vi "BC Test - Messages Only.vi"() -> ()   [LabVIEW 2016]
uses:
  Bus Controller/TypeDefs/Bus Controller Configuration.ctl
  Frames & Messages/TypeDefs/Message Config.ctl
  Frames & Messages/TypeDefs/Command Config.ctl
  Frames & Messages/TypeDefs/Message Control.ctl
  1553 SubComponent/TypeDefs/Parameter Table Data.ctl
  1553 SubComponent/TypeDefs/Scaling Information.ctl
  Frames & Messages/TypeDefs/RT-RT Message Config.ctl
  1553 Board/1553 Board.lvclass/1553 Board.ctl
  Bus Controller/Bus Controller.lvclass
  C:/SLSC 1553/Driver (Windows)/1553 SubComponent/1553 SubComponent.lvclass
  Frames & Messages/Message/Message.lvclass
  1553 Component/1553 Component.lvclass
  Frames & Messages/Major Frame/Major Frame.lvclass
  1553 Board/1553 Board.lvclass
  Utilities/FPGA Interface/FPGA Interface.lvclass
  SLSC 1553 API.lvlib
  1553 SubComponent/1553 SubComponent.lvclass
  Frames & Messages/RT-RT Message/RT-RT Message.lvclass
  C:/SLSC 1553/Driver (Windows)/Frames & Messages/Message/Message.lvclass
panel:
  in  "Inhibit Bus B":bool
  in  "Inhibit Bus A":bool
  in  "Scaled Data 2":dbl[](array[numeric])
  in  "Parameters 2":string[](array[string])
  in  "Update Param":bool
  out "Scaled Data":dbl[][](array[numeric])
  out "Parameters":string[][](array[string])
  out "error out":errorcluster
  in  "stop":bool
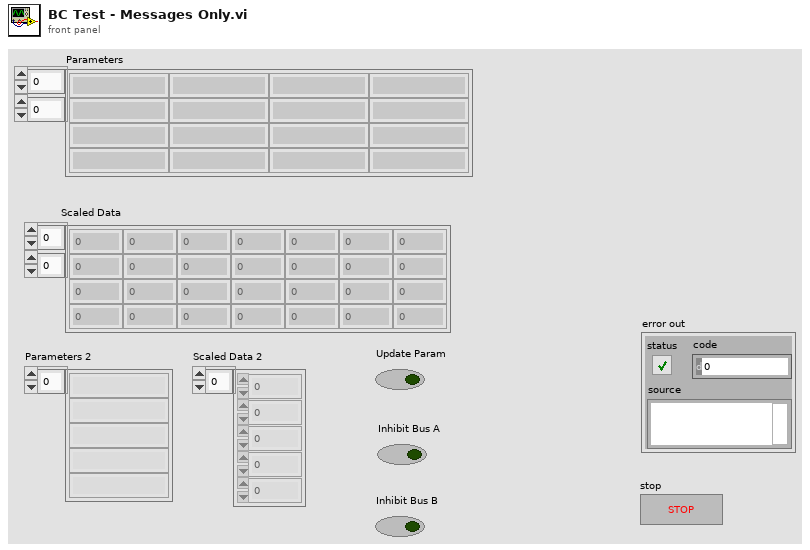
[diagram p1: front panel]
types:
  T1 = typedef "SLSC 1553 API.lvlib/RT-RT Message Config.ctl" = cluster{"Tx Command Config":T2}
  T2 = typedef "SLSC 1553 API.lvlib/Command Config.ctl" = cluster{"Command Type":enum16{"Transmit", "Receive"}, "Terminal Address (0-30)":u16, "SubAddress (1-30)":u16, "WC/MC (1-32)":u16, "Command Data":u16[]}
  T3 = typedef "SLSC 1553 API.lvlib/1553 SubComponent.lvclass/Parameter Table Data.ctl" = cluster{"Parameter Name":string, "Base Word":u16, "Address":u16, "Value":u64, "Mask":u16[], "Scaling Info":T4}
  T4 = typedef "SLSC 1553 API.lvlib/1553 SubComponent.lvclass/Scaling Information.ctl" = cluster{"Bit Offset":i32, "Bit Count":i32, "LSB Resolution":dbl, "2's Complement":bool, "Big Endian":bool}
  T5 = typedef "SLSC 1553 API.lvlib/Message Config.ctl" = cluster{"Time to Next Msg (100 us)":u16, "Command Config":T2, "Message Control":T6}
  T6 = typedef "SLSC 1553 API.lvlib/Message Control.ctl" = cluster{"MC17 Time Sync":bool, "Error Mask":bool, "Service Request Mask":bool, "Busy Mask":bool, "SubSystem Flag Mask":bool, "Terminal Flag Mask":bool, "Reserved Mask":bool, "Retry":bool, "Bus A / !Bus B":bool, "Self-Test Loopback":bool, "Broadcast Mask":bool, "EoM Interrupt":bool, "Mode Code Format":bool, "Broadcast Format":bool, "RT-RT Format":bool}
  T7 = typedef "SLSC 1553 API.lvlib/Bus Controller.lvclass/Bus Controller Configuration.ctl" = cluster{"BC Timeout":u16, "BC Retry":bool, "BC Second Retry":bool, "BC Retry Alt Bus":bool, "BC Second Retry Alt Bus":bool, "BC Retry on Status Bit":bool, "Msg Error No Data Valid":bool, "Busy Status No Data Valid":bool, "Msg Gap Timer":bool, "Watchdog Timer":bool, "Time Tag Sync":bool, "Even Time Tag Sync":bool, "Gap Check":bool, "Broadcast Mask Enable":bool}
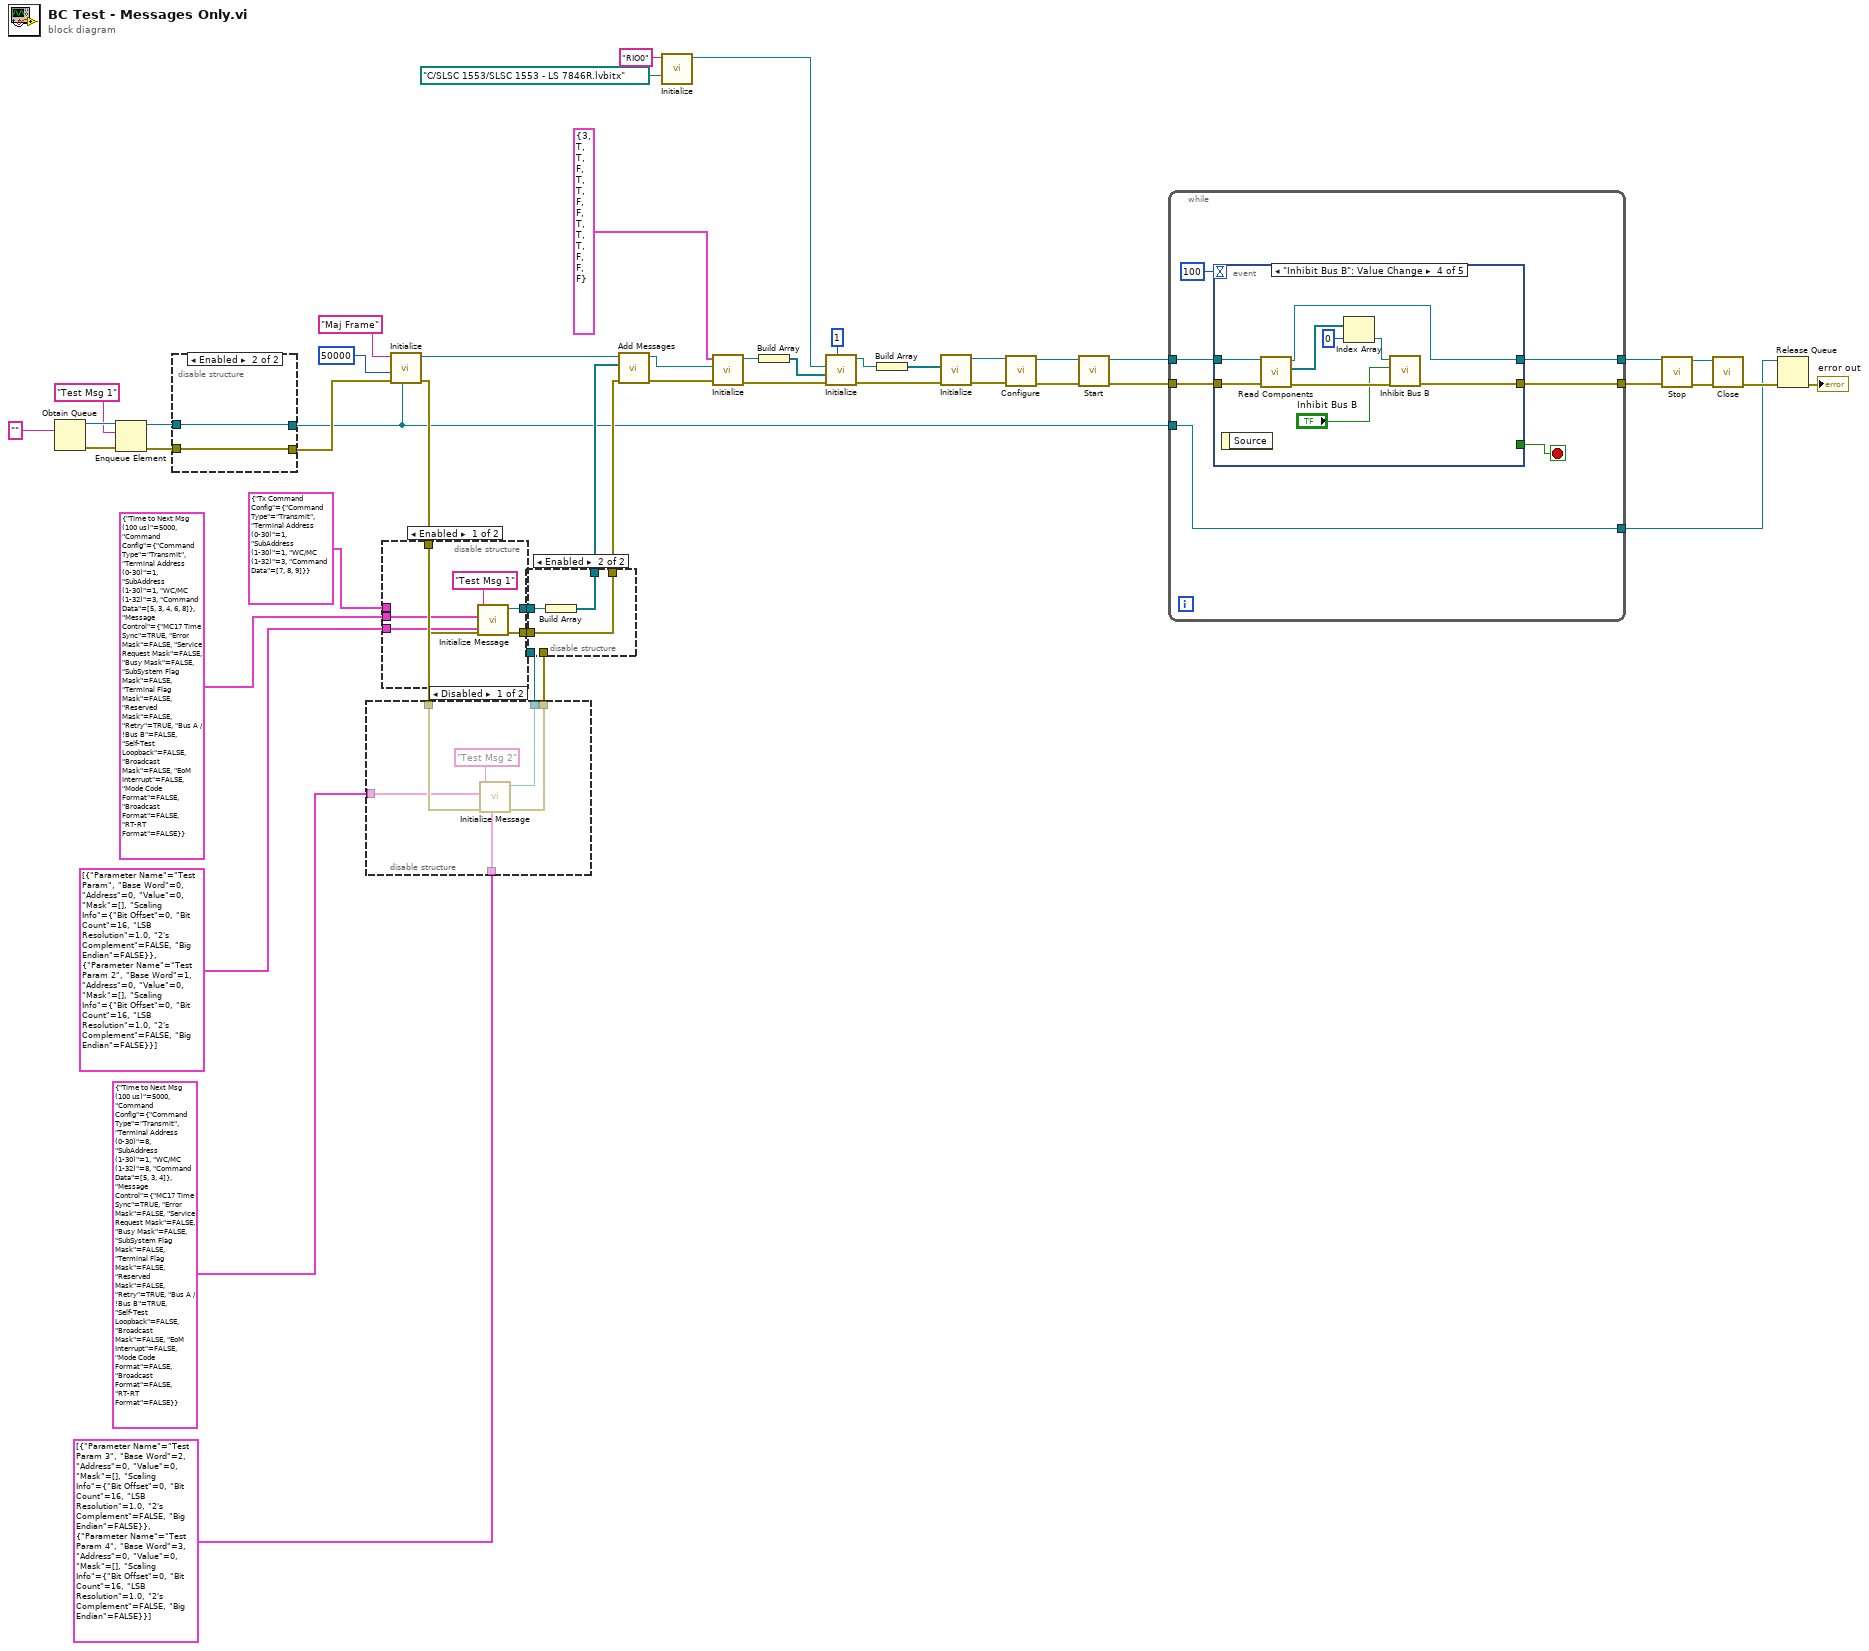
[diagram p0: block diagram]
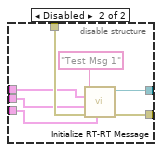
[diagram p2: hidden frame]
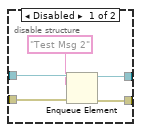
[diagram p3: hidden frame]
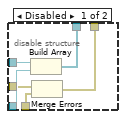
[diagram p4: hidden frame]
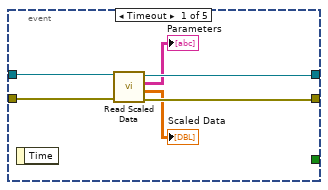
[diagram p6: hidden frame]
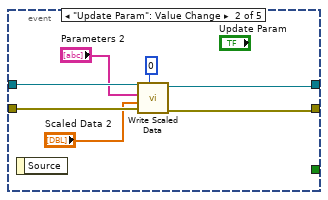
[diagram p7: hidden frame]
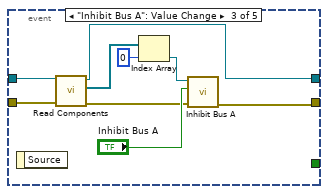
[diagram p8: hidden frame]
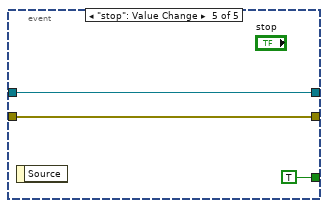
[diagram p9: hidden frame]
diagram:
  n1 = Obtain Queue(element data type="") -> (queue out=w46:refnum<queue>, error out=w47:errorcluster)  [unwired: 4 in, 1 out]
  n2 = Enqueue Element(queue=w46, element="Test Msg 1", error in (no error)=w47) -> (queue out=w44:refnum<queue>, error out=w45:errorcluster)  [unwired: 1 in, 1 out]
  n3 = disable-structure shown="Enabled" {
    disable-tunnel: w45 -> [w54 w55]
    disable-tunnel: w44 -> [w53 w56]
    disable-tunnel: [w51 w55] -> w42
    disable-tunnel: [w50 w56] -> w4
    frame Disabled {
      n4 = Enqueue Element(queue=w53, element="Test Msg 2", error in (no error)=w54) -> (queue out=w50:refnum<queue>, error out=w51:errorcluster)  [unwired: 1 in, 1 out]
    }
    frame Enabled {
    }
  }
  n5 = call "Initialize.vi"("Schedule"=w4, "error in (no error)"=w42, "Minor Frame Time (us)"=u16 50000, "ID"="Maj Frame") -> ("error out"=w40:errorcluster, "Major Frame out"=w41:refnum<class "Major Frame.lvclass">)  [unwired: 6 in]
  n6 = disable-structure shown="Disabled" {
    disable-tunnel: w40 -> [w61 _]
    disable-tunnel: [w60 _] -> w38
    disable-tunnel: [w59 _] -> w33
    disable-tunnel: T5 {"Time to Next Msg (100 us)"=5000, "Command Config"={"Command Type"=enum."Transmit", "Terminal Address (0-30)"=8, "SubAddress (1-30)"=1, "WC/MC (1-32)"=8, "Command Data"=[5, 3, 4]}, "Message Control"={"MC17 Time Sync"=TRUE, "Error Mask"=FALSE, "Service Request Mask"=FALSE, "Busy Mask"=FALSE, "SubSystem Flag Mask"=FALSE, "Terminal Flag Mask"=FALSE, "Reserved Mask"=FALSE, "Retry"=TRUE, "Bus A / !Bus B"=TRUE, "Self-Test Loopback"=FALSE, "Broadcast Mask"=FALSE, "EoM Interrupt"=FALSE, "Mode Code Format"=FALSE, "Broadcast Format"=FALSE, "RT-RT Format"=FALSE}} ("Message  Config") -> [w58 _]
    disable-tunnel: T3[] [{"Parameter Name"="Test Param 3", "Base Word"=2, "Address"=0, "Value"=0, "Mask"=[], "Scaling Info"={"Bit Offset"=0, "Bit Count"=16, "LSB Resolution"=1.0, "2's Complement"=FALSE, "Big Endian"=FALSE}}, {"Parameter Name"="Test Param 4", "Base Word"=3, "Address"=0, "Value"=0, "Mask"=[], "Scaling Info"={"Bit Offset"=0, "Bit Count"=16, "LSB Resolution"=1.0, "2's Complement"=FALSE, "Big Endian"=FALSE}}] ("Parameters") -> [w57 _]
    frame Disabled {
      n7 = call "Initialize Message.vi"("Parameters"=w57, "error in (no error)"=w61, "Message  Config"=w58, "ID"="Test Msg 2") -> ("error out"=w59:errorcluster, "Message out"=w60:refnum<class "Message.lvclass">)  [unwired: 6 in]
    }
    frame Enabled {
    }
  }
  n8 = disable-structure shown="Enabled" {
    disable-tunnel: w40 -> [w67 w73]
    disable-tunnel: [w66 w74] -> w39
    disable-tunnel: [w65 w75] -> w34
    disable-tunnel: T5 {"Time to Next Msg (100 us)"=5000, "Command Config"={"Command Type"=enum."Transmit", "Terminal Address (0-30)"=1, "SubAddress (1-30)"=1, "WC/MC (1-32)"=3, "Command Data"=[5, 3, 4, 6, 8]}, "Message Control"={"MC17 Time Sync"=TRUE, "Error Mask"=FALSE, "Service Request Mask"=FALSE, "Busy Mask"=FALSE, "SubSystem Flag Mask"=FALSE, "Terminal Flag Mask"=FALSE, "Reserved Mask"=FALSE, "Retry"=TRUE, "Bus A / !Bus B"=FALSE, "Self-Test Loopback"=FALSE, "Broadcast Mask"=FALSE, "EoM Interrupt"=FALSE, "Mode Code Format"=FALSE, "Broadcast Format"=FALSE, "RT-RT Format"=FALSE}} ("Message  Config") -> [w64 w70]
    disable-tunnel: T3[] [{"Parameter Name"="Test Param", "Base Word"=0, "Address"=0, "Value"=0, "Mask"=[], "Scaling Info"={"Bit Offset"=0, "Bit Count"=16, "LSB Resolution"=1.0, "2's Complement"=FALSE, "Big Endian"=FALSE}}, {"Parameter Name"="Test Param 2", "Base Word"=1, "Address"=0, "Value"=0, "Mask"=[], "Scaling Info"={"Bit Offset"=0, "Bit Count"=16, "LSB Resolution"=1.0, "2's Complement"=FALSE, "Big Endian"=FALSE}}] ("Parameters") -> [w63 w69]
    disable-tunnel: T1 {"Tx Command Config"={"Command Type"=enum."Transmit", "Terminal Address (0-30)"=1, "SubAddress (1-30)"=1, "WC/MC (1-32)"=3, "Command Data"=[7, 8, 9]}} ("RT-RT Message Config") -> [_ w71]
    frame Enabled {
      n9 = call "Initialize Message.vi"("Parameters"=w63, "error in (no error)"=w67, "Message  Config"=w64, "ID"="Test Msg 1") -> ("error out"=w65:errorcluster, "Message out"=w66:refnum<class "Message.lvclass">)  [unwired: 6 in]
    }
    frame Disabled {
      n10 = call "Initialize RT-RT Message.vi"("Parameters"=w69, "error in (no error)"=w73, "Message Config"=w70, "RT-RT Message Config"=w71, "ID"="Test Msg 1") -> ("error out"=w75:errorcluster, "RT-RT Message out"=w74:refnum<class "RT-RT Message.lvclass">)  [unwired: 5 in]
    }
  }
  n11 = disable-structure shown="Enabled" {
    disable-tunnel: w39 -> [w81 w84]
    disable-tunnel: w38 -> [w80 _]
    disable-tunnel: [w79 w83] -> w37
    disable-tunnel: w34 -> [w78 w82]
    disable-tunnel: w33 -> [w77 _]
    disable-tunnel: [w76 w82] -> w32
    frame Disabled {
      n12 = Build Array(w81, w80) -> (w79:refnum<class "Message.lvclass">[])
      n13 = Merge Errors(w78, w77) -> (w76:errorcluster)
    }
    frame Enabled {
      n14 = Build Array(w84) -> (w83:refnum<class "Message.lvclass">[])
    }
  }
  n15 = call-dynamic "Add Messages.vi"("error in (no error)"=w32, "Messages"=w37, "Major Frame in"=w41) -> ("error out"=w35:errorcluster, "Major Frame out"=w36:refnum<class "Major Frame.lvclass">)  [unwired: 7 in]
  n16 = call "Initialize.vi"("Bitfile path"=path "C:/SLSC 1553/SLSC 1553 - LS 7846R.lvbitx", "Device address"="RIO0") -> ("FPGA Interface out"=w24:refnum<class "FPGA Interface.lvclass">)  [unwired: 8 in, 1 out]
  n17 = call "Initialize.vi"("error in (no error)"=w35, "Major Frame"=w36, "Configuration"=T7 {"BC Timeout"=3, "BC Retry"=TRUE, "BC Second Retry"=TRUE, "BC Retry Alt Bus"=FALSE, "BC Second Retry Alt Bus"=TRUE, "BC Retry on Status Bit"=TRUE, "Msg Error No Data Valid"=FALSE, "Busy Status No Data Valid"=FALSE, "Msg Gap Timer"=TRUE, "Watchdog Timer"=TRUE, "Time Tag Sync"=TRUE, "Even Time Tag Sync"=FALSE, "Gap Check"=FALSE, "Broadcast Mask Enable"=FALSE}) -> ("error out"=w28:errorcluster, "Bus Controller out"=w26:refnum<class "Bus Controller.lvclass">)  [unwired: 7 in]
  n18 = Build Array(w26) -> (w25:refnum<class "Bus Controller.lvclass">[])
  n19 = call "Initialize.vi"("Component ID (1-8)"=u8 1, "error in (no error)"=w28, "SubComponents"=w25, "FPGA Interface"=w24) -> ("error out"=w23:errorcluster, "1553 Component out"=w22:refnum<class "1553 Component.lvclass">)  [unwired: 6 in]
  n20 = Build Array(w22) -> (w21:refnum<class "1553 Component.lvclass">[])
  n21 = call "Initialize.vi"("error in (no error)"=w23, "Components"=w21) -> ("error out"=w16:errorcluster, "1553 Board out"=w15:refnum<class "1553 Board.lvclass">)  [unwired: 8 in]
  n22 = call-dynamic "Configure.vi"("error in (no error)"=w16, "1553 Board in"=w15) -> ("error out"=w14:errorcluster, "1553 Board out"=w13:refnum<class "1553 Board.lvclass">)  [unwired: 8 in]
  n23 = call-dynamic "Start.vi"("error in (no error)"=w14, "1553 Board in"=w13) -> ("error out"=w12:errorcluster, "1553 Board out"=w11:refnum<class "1553 Board.lvclass">)  [unwired: 8 in]
  n24 = while {
    tunnel: w12 -> [w90]
    tunnel: w11 -> [w89]
    tunnel: [w87] -> w10
    tunnel: [w86] -> w9
    tunnel: w4 -> [w85]
    tunnel: [w85] -> w3
    stop <- w88 stop-if-true
    n25 = event shown="[3] \"Inhibit Bus B\": Value Change" {
      selector: _ -> [_ _ _ _ _]
      dyn-events: _ -> [_ _ _ _ _]
      timeout: 100 -> [_ _ _ _ _]
      tunnel: w90 -> [w97 w104 w113 w122 w124]
      tunnel: w89 -> [w96 w103 w112 w121 w123]
      tunnel: [_ _ _ _ TRUE] -> w88
      tunnel: [w95 w100 w106 w115 w124] -> w87
      tunnel: [w94 w101 w105 w118 w123] -> w86
      event Timeout {
        n26 = event-data() -> ()  [unwired: 1 in, 1 out]
        n27 = call-dynamic "Read Scaled Data.vi"("error in (no error)"=w97, "1553 Board in"=w96) -> ("error out"=w95:errorcluster, "Scaled Data"=→"Scaled Data":dbl[][], "Parameters"=→"Parameters":string[][], "1553 Board out"=w94:refnum<class "1553 Board.lvclass">)  [unwired: 6 in]
      }
      event "Update Param": Value Change {
        n28 = event-data() -> ()  [unwired: 1 in, 1 out]
        n29 = call-dynamic "Write Scaled Data.vi"("Component Index"=0, "error in (no error)"=w104, "Scaled Data"="Scaled Data 2", "Parameters"="Parameters 2", "1553 Board in"=w103) -> ("error out"=w100:errorcluster, "1553 Board out"=w101:refnum<class "1553 Board.lvclass">)  [unwired: 5 in]
      }
      event "Inhibit Bus A": Value Change {
        n30 = event-data() -> ()  [unwired: 1 in, 1 out]
        n31 = call "Read Components.vi"("error in (no error)"=w113, "1553 Board in"=w112) -> ("error out"=w107:errorcluster, "Components"=w111:refnum<class "1553 Component.lvclass">[], "1553 Board out"=w105:refnum<class "1553 Board.lvclass">)  [unwired: 7 in]
        n32 = Index Array(array=w111, index=0) -> (element=w109:refnum<class "1553 Component.lvclass">)
        n33 = call-dynamic "Inhibit Bus A.vi"("error in (no error)"=w107, "Inhibit Bus A?"="Inhibit Bus A", "1553 Component in"=w109) -> ("error out"=w106:errorcluster)  [unwired: 8 in]
      }
      event "Inhibit Bus B": Value Change {
        n34 = event-data() -> ()  [unwired: 1 in, 1 out]
        n35 = call "Read Components.vi"("error in (no error)"=w122, "1553 Board in"=w121) -> ("error out"=w117:errorcluster, "Components"=w120:refnum<class "1553 Component.lvclass">[], "1553 Board out"=w118:refnum<class "1553 Board.lvclass">)  [unwired: 7 in]
        n36 = Index Array(array=w120, index=0) -> (element=w116:refnum<class "1553 Component.lvclass">)
        n37 = call-dynamic "Inhibit Bus B.vi"("error in (no error)"=w117, "Inhibit Bus B?"="Inhibit Bus B", "1553 Component in"=w116) -> ("error out"=w115:errorcluster)  [unwired: 8 in]
      }
      event "stop": Value Change {
        n38 = event-data() -> ()  [unwired: 1 in, 1 out]
      }
    }
  }
  n39 = call-dynamic "Stop.vi"("error in (no error)"=w10, "1553 Board in"=w9) -> ("error out"=w8:errorcluster, "1553 Board out"=w7:refnum<class "1553 Board.lvclass">)  [unwired: 8 in]
  n40 = call-dynamic "Close.vi"("error in (no error)"=w8, "1553 Board in"=w7) -> ("error out"=w6:errorcluster)  [unwired: 9 in]
  n41 = Release Queue(queue=w3, error in (no error)=w6) -> (error out=→"error out":errorcluster)  [unwired: 1 in, 2 out]
